vi "Integration Start Stop.vi"(9 "Element (All: 0)":T1(ring), 10 "Start/Stop (F: Stop)":bool, 11 "WT1600.lvlib:WT1600.lvclass":refnum<class "WT1600.lvclass">) -> (3 "WT1600 out":refnum<class "WT1600.lvclass">)   [LabVIEW 2013, in "Universal Power Meter.lvlib" / "WT1600.lvlib" / "WT1600.lvclass"]
uses:
  WT1600.lvclass
  WT1600.lvclass/WT1600.ctl
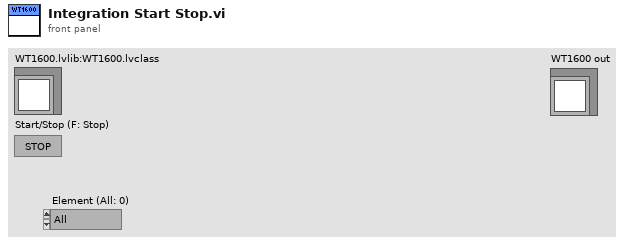
[diagram p1: front panel]
types:
  T1 = enum16{"All", "Element 1", "Element 2", "Element 3", "Element 4", "Element 5", "Element 6"}
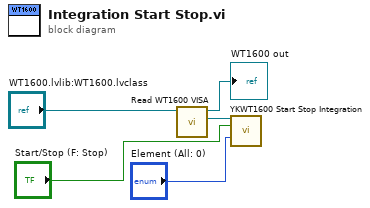
[diagram p0: block diagram]
diagram:
  n1 = call "Read WT1600 VISA.vi"("WT1600 in"="WT1600.lvlib:WT1600.lvclass") -> ("WT1600 VISA"=w3:refnum<visa-resource-name>, "WT1600 out"=→"WT1600 out":refnum<class "WT1600.lvclass">)  [unwired: 8 in, 1 out]
  n2 = call <instrlib>:"YKWT1600 Start Stop Integration.vi"("VISA session"=w3, "Start/Stop (F: Stop)"="Start/Stop (F: Stop)", "Element (All: 0)"="Element (All: 0)") -> ()  [unwired: 11 in, 2 out]
